vi "rmad skredstorrelse.vi"(0 "Is Logging":T5(array[cluster]), 1 "State":u16(ring) items=["Init", "Write"], 2 "Rød signal kriterie":bool[](array[boolean]), 5 "Avalanch Packets":T4(array[cluster]) {"A1 std" format="%.1f"; "A2 std" format="%.1f"; "A3 std" format="%.1g"; "A4 std" format="%.1g"}, 7 "Recent events":T1(array[cluster]) {"SPS" format="%.1f"}, 12 "Stredstørrelser terskelverdier":T2(array[cluster])) -> (4 "Skredhendelser":T3(array[cluster]) {"Intensitet terskel 1" format="%.1f"; "Intensitet terskel 2" format="%.1f"; "Intensitet terskel 3" format="%.1f"; "Intensitet terskel 4" format="%.1f"; "Intensitet terskel 5" format="%.1f"}, 6 "event to regobs":bool[](array[boolean]), 8 "event to file?":bool[](array[boolean]), 10 "is logging":bool[](array[boolean]), 14 "num pack pr size":u16[][](array[numeric]))   [LabVIEW 2017]
panel:
  out "har aktivert rødt lys":bool[](array[boolean])
  out "løpende gjennomsnitt":dbl[][](array[numeric])
  out "sum intensiteter":dbl[][](array[numeric])
  out "har trigget på denne event":bool[](array[boolean])
  out "skredstorelse index":i32[](array[numeric])
  out "packet number index":u16[](array[numeric])
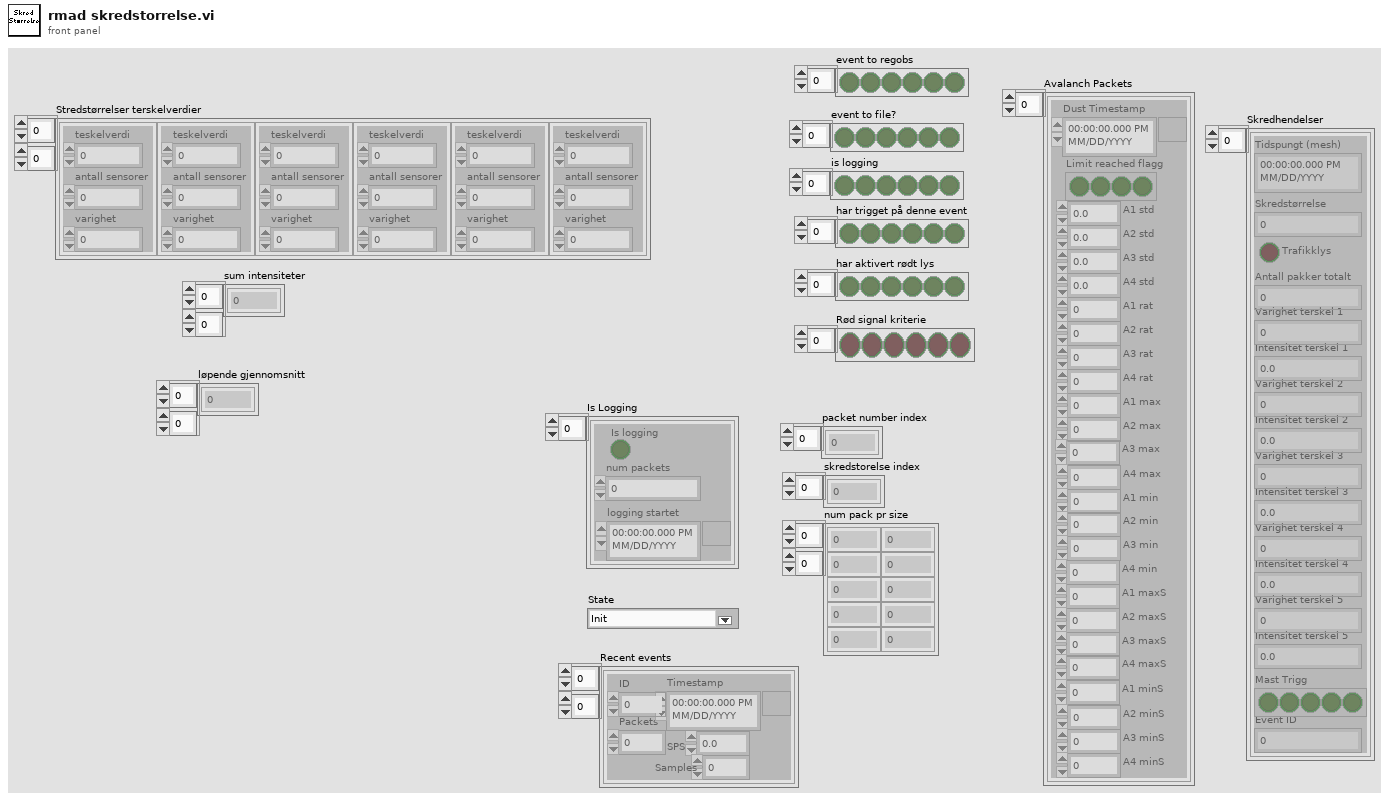
[diagram p1: front panel]
types:
  T1 = cluster{"ID":u16, "Timestamp":timestamp, "Packets":u16, "SPS":dbl, "Samples":u16}[][]
  T2 = cluster{"teskelverdi":u32, "antall sensorer":u32, "varighet":u32}[][]
  T3 = cluster{"Tidspungt (mesh)":timestamp, "Skredstørrelse":u16, "Trafikklys":bool, "Antall pakker totalt":u16, "Varighet terskel 1":u16, "Intensitet terskel 1":dbl, "Varighet terskel 2":u16, "Intensitet terskel 2":dbl, "Varighet terskel 3":u16, "Intensitet terskel 3":dbl, "Varighet terskel 4":u16, "Intensitet terskel 4":dbl, "Varighet terskel 5":u16, "Intensitet terskel 5":dbl, "Mast Trigg":bool[], "Event ID":i32}[]
  T4 = cluster{"Dust Timestamp":timestamp, "Limit reached flagg":bool[], "A1 std":sgl, "A2 std":sgl, "A3 std":sgl, "A4 std":sgl, "A1 rat":sgl, "A2 rat":sgl, "A3 rat":sgl, "A4 rat":sgl, "A1 max":u16, "A2 max":u16, "A3 max":u16, "A4 max":u16, "A1 min":u16, "A2 min":u16, "A3 min":u16, "A4 min":u16, "A1 maxS":u16, "A2 maxS":u16, "A3 maxS":u16, "A4 maxS":u16, "A1 minS":u16, "A2 minS":u16, "A3 minS":u16, "A4 minS":u16}[]
  T5 = cluster{"Is logging":bool, "num packets":u16, "logging startet":timestamp}[]
  T6 = cluster{"logging startet":timestamp, i32, bool, "num packets":u16, u16, dbl, u16, dbl, u16, dbl, u16, dbl, u16, dbl, bool[], "index":i32}
  T7 = cluster{"ID":u16, "Timestamp":timestamp, "Packets":u16, "SPS":dbl, "Samples":u16}
  T8 = cluster{"logging startet":timestamp, i32, bool, "num packets":u16, u16, dbl, u16, dbl, "index":i32, "index":i32, "index":i32, "index":i32, "index":i32, "index":i32, bool[], "ID":u16}
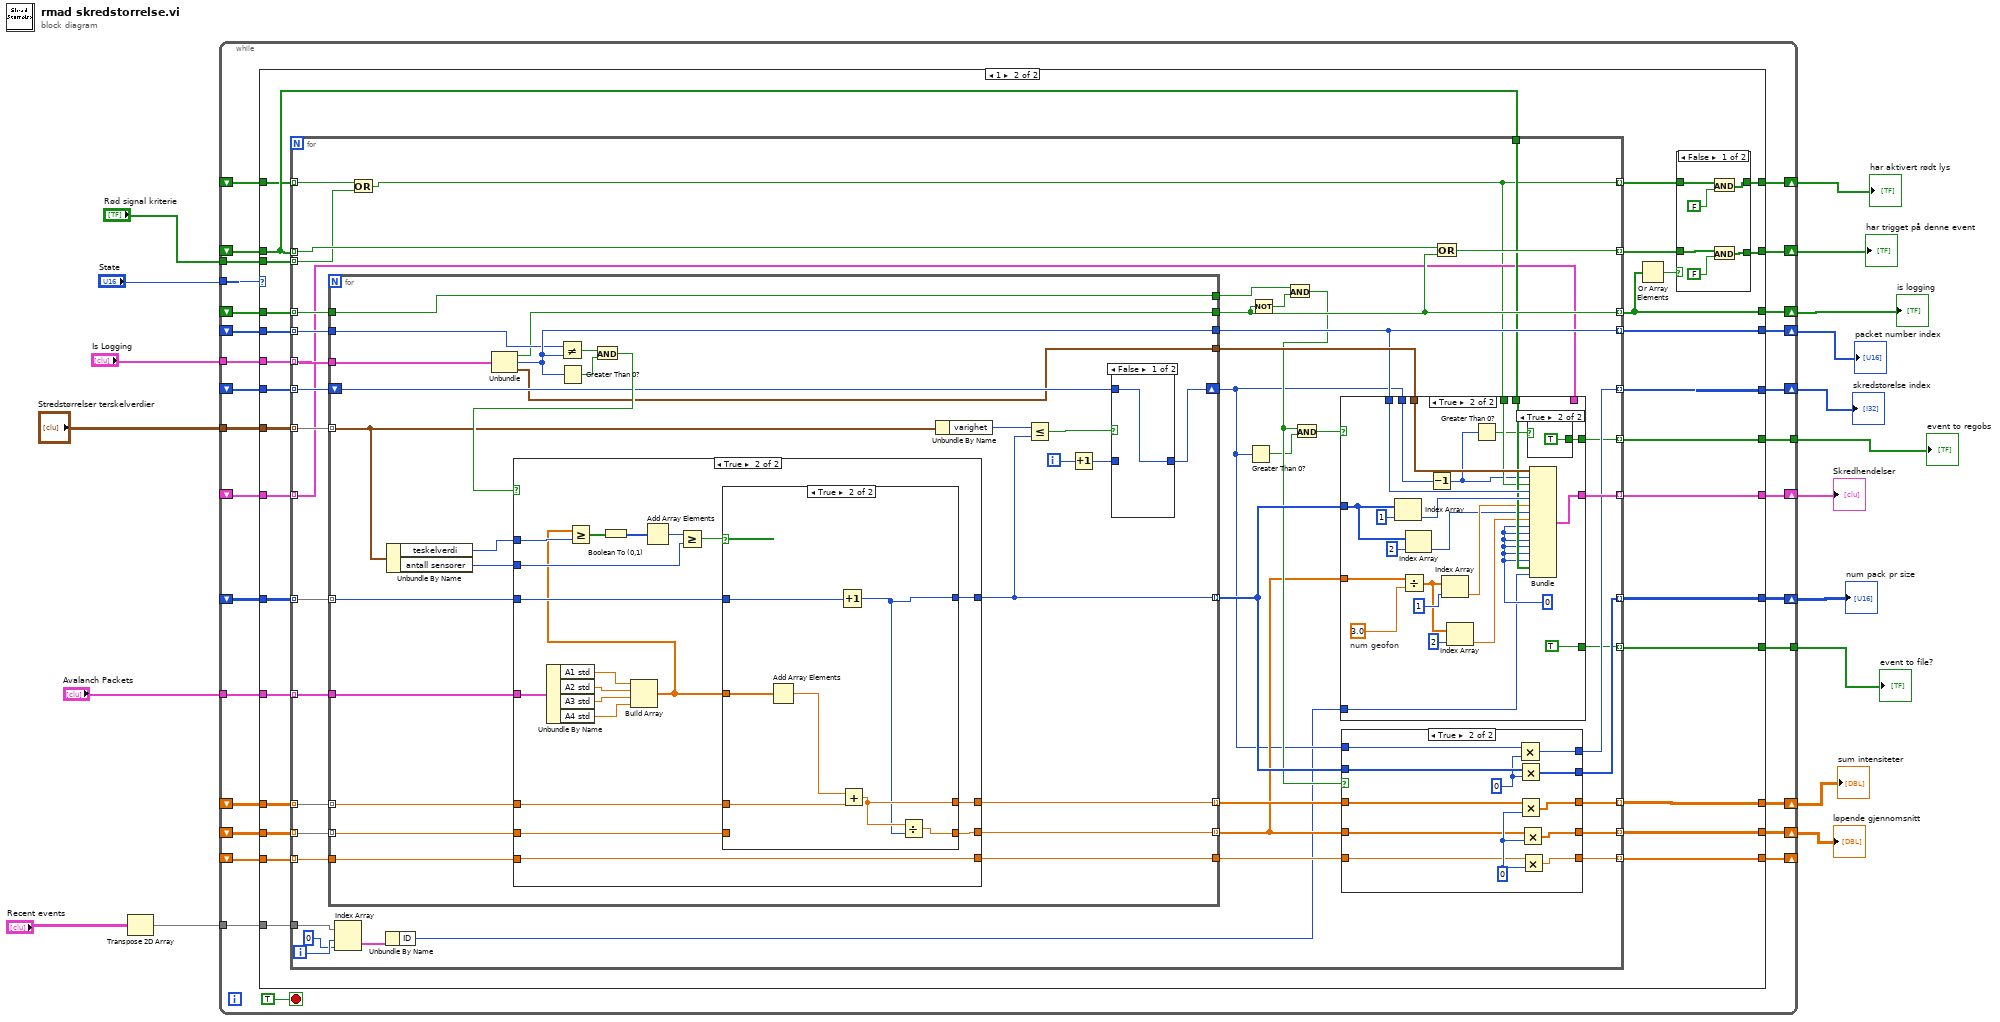
[diagram p0: block diagram]
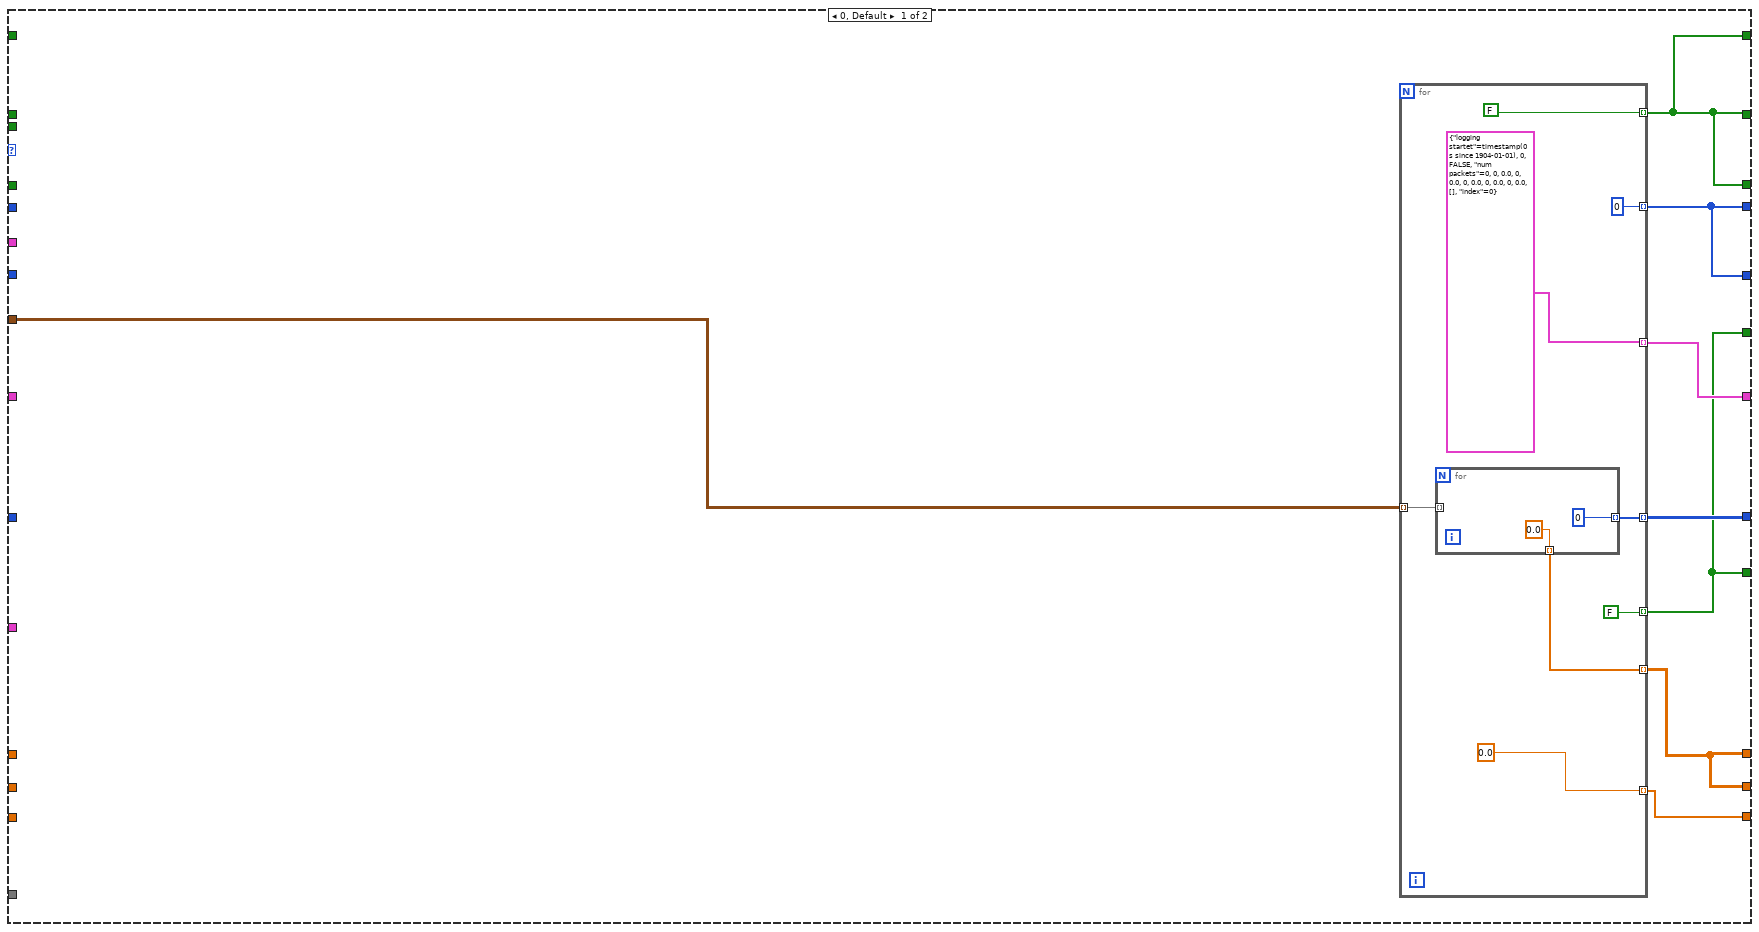
[diagram p2: hidden frame]
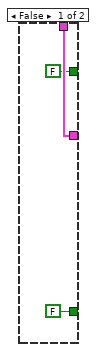
[diagram p5: hidden frame]
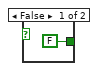
[diagram p6: hidden frame]
diagram:
  n1 = Transpose 2D Array(2D array="Recent events") -> (transposed array=w4:T1)
  n2 = while {
    tunnel: "Is Logging" -> [w47]
    tunnel: "Avalanch Packets" -> [w45]
    tunnel: "State" -> [w44]
    tunnel: "Stredstørrelser terskelverdier" -> [w43]
    shift-right: [w42] -> w11
    shift-left: _ -> [w41]
    shift-right: [w40] -> w15
    shift-left: _ -> [w39]
    shift-right: [w38] -> w14
    shift-left: _ -> [w37]
    shift-right: [w36] -> _
    shift-left: _ -> [w33]
    shift-right: [w35] -> w8
    shift-left: _ -> [w32]
    shift-right: [w34] -> w10
    shift-left: _ -> [w31]
    shift-right: [w30] -> w13
    shift-left: _ -> [w29]
    shift-right: [w28] -> w12
    shift-left: _ -> [w27]
    shift-right: [w26] -> w9
    shift-left: _ -> [w25]
    tunnel: [w24] -> w6
    tunnel: "Rød signal kriterie" -> [w23]
    tunnel: w4 -> [w22]
    tunnel: [w21] -> w2
    shift-right: [w20] -> w1
    shift-left: _ -> [w19]
    stop <- TRUE stop-if-true
    n3 = case shown="1" w44 {
      tunnel: w47 -> [_ w95]
      tunnel: w45 -> [_ w94]
      tunnel: w43 -> [w54 w93]
      tunnel: [w53 w92] -> w42
      tunnel: w41 -> [_ w91]
      tunnel: [w55 w90] -> w40
      tunnel: w39 -> [_ w89]
      tunnel: [w55 w88] -> w38
      tunnel: w37 -> [_ w87]
      tunnel: [w51 w86] -> w36
      tunnel: [w50 w85] -> w35
      tunnel: [w50 w84] -> w34
      tunnel: w33 -> [_ w83]
      tunnel: w32 -> [_ w82]
      tunnel: w31 -> [_ w81]
      tunnel: [w48 w79] -> w30
      tunnel: w29 -> [_ w80]
      tunnel: [w48 w77] -> w28
      tunnel: w27 -> [_ w75]
      tunnel: [w52 w74] -> w26
      tunnel: w25 -> [_ w73]
      tunnel: [w49 w72] -> w24
      tunnel: w23 -> [_ w71]
      tunnel: w22 -> [_ w70]
      tunnel: [w49 w69] -> w21
      tunnel: [w48 w66] -> w20
      tunnel: w19 -> [_ w68]
      frame 0, Default {
        n4 = for {
          tunnel: [u16 0] -> w55 mode=indexing
          tunnel: [FALSE] -> w48 mode=indexing
          tunnel: [0.0 ("number")] -> w51 mode=indexing
          tunnel: w54 -> [w60] mode=indexing
          tunnel: [w59] -> w53 mode=indexing
          tunnel: [T6 {"logging startet"=timestamp(0 s since 1904-01-01), 0, FALSE, "num packets"=0, 0, 0.0, 0, 0.0, 0, 0.0, 0, 0.0, 0, 0.0, [], "index"=0}] -> w52 mode=indexing
          tunnel: [w58] -> w50 mode=indexing
          tunnel: [FALSE] -> w49 mode=indexing
          n5 = for {
            tunnel: w60 -> [_] mode=indexing
            tunnel: [u16 0] -> w59 mode=indexing
            tunnel: [0.0 ("number")] -> w58 mode=indexing
          }
        }
      }
      frame 1 {
        n6 = for {
          tunnel: w95 -> [w145] mode=indexing
          tunnel: w94 -> [w146] mode=indexing
          tunnel: w93 -> [w144] mode=indexing
          tunnel: [w122] -> w92 mode=indexing
          tunnel: w91 -> [w143] mode=indexing
          tunnel: [w133] -> w90 mode=indexing
          tunnel: w89 -> [w142] mode=indexing
          tunnel: [w116] -> w88 mode=indexing
          tunnel: w87 -> [w141] mode=indexing
          tunnel: [w125] -> w86 mode=indexing
          tunnel: [w124] -> w85 mode=indexing
          tunnel: [w123] -> w84 mode=indexing
          tunnel: w83 -> [w140] mode=indexing
          tunnel: w82 -> [w139] mode=indexing
          tunnel: w81 -> [w138] mode=indexing
          tunnel: [w132] -> w79 mode=indexing
          tunnel: w80 -> [w137] mode=indexing
          tunnel: [w131] -> w78 mode=indexing
          tunnel: w75 -> [w130] mode=indexing
          tunnel: w75 -> [w129]
          tunnel: [w128] -> w74 mode=indexing
          tunnel: w73 -> [w127] mode=indexing
          tunnel: [w114] -> w72 mode=indexing
          tunnel: w71 -> [w105] mode=indexing
          tunnel: w70 -> [w113]
          tunnel: [w107] -> w69 mode=indexing
          tunnel: w68 -> [w106] mode=indexing
          tunnel: [w104] -> w67 mode=indexing
          i -> [w110]
          n7 = for {
            tunnel: w146 -> [w218]
            tunnel: w145 -> [w215]
            tunnel: w144 -> [w209] mode=indexing
            tunnel: [w195] -> w126 mode=indexing
            tunnel: w143 -> [w214] mode=indexing
            tunnel: [w211] -> w133
            tunnel: w142 -> [w210]
            shift-right: [w204] -> w117
            shift-left: w141 -> [w203]
            tunnel: [w202] -> w121
            tunnel: [w201] -> w118 mode=indexing
            tunnel: [w200] -> w119 mode=indexing
            tunnel: w140 -> [w199]
            tunnel: w139 -> [w198] mode=indexing
            tunnel: w138 -> [w197] mode=indexing
            tunnel: [w196] -> w132
            tunnel: w137 -> [w194]
            tunnel: [w194] -> w135
            tunnel: [w193] -> w134
            i -> [w206]
            n8 = Unbundle By Name(w209) -> ("teskelverdi"=w216:u32, "antall sensorer"=w217:u32)
            n9 = Unbundle(w215) -> ("Is logging"=w196:bool, "num packets"=w211:u16, "logging startet"=w193:timestamp)
            n10 = Not Equal?(x=w210, y=w211) -> (x != y?=w219:bool)
            n11 = Greater Than 0?(x=w211) -> (x > 0?=w213:bool)
            n12 = And(x=w219, y=w213) -> (x .and. y?=w212:bool)
            n13 = case shown="True" w212 {
              tunnel: w218 -> [_ w244]
              tunnel: w217 -> [_ w234]
              tunnel: w216 -> [_ w235]
              tunnel: [w225 w233] -> w195
              tunnel: w214 -> [w225 w232]
              tunnel: [w222 w230] -> w202
              tunnel: [w223 w227] -> w201
              tunnel: [w224 w228] -> w200
              tunnel: w199 -> [w222 w230]
              tunnel: w198 -> [w223 w226]
              tunnel: w197 -> [w224 w229]
              frame False {
              }
              frame True {
                n14 = Unbundle By Name(w244) -> ("A1 std"=w242:sgl, "A2 std"=w243:sgl, "A3 std"=w241:sgl, "A4 std"=w240:sgl)
                n15 = Build Array(w242, w243, w241, w240) -> (w231:sgl[])
                n16 = Greater Or Equal?(x=w231, y=w235) -> (x >= y?=w239:bool[])
                n17 = Boolean To (0,1)(Boolean=w239) -> (0, 1=w238:i16[])
                n18 = Add Array Elements(numeric array=w238) -> (sum=w237:i16)
                n19 = Greater Or Equal?(x=w237, y=w234) -> (x >= y?=w236:bool)
                n20 = case shown="True" w236 {
                  tunnel: [w247 w249] -> w233
                  tunnel: w232 -> [w247 w254]
                  tunnel: w231 -> [_ w253]
                  tunnel: w229 -> [w246 w252]
                  tunnel: [w246 w250] -> w228
                  tunnel: [w245 w248] -> w227
                  tunnel: w226 -> [w245 _]
                  frame False {
                  }
                  frame True {
                    n21 = Add Array Elements(numeric array=w253) -> (sum=w251:sgl)
                    n22 = Increment(x=w254) -> (x+1=w249:u16)
                    n23 = Add(x=w251, y=w252) -> (x+y=w250:dbl)
                    n24 = Divide(x=w250, y=w249) -> (x/y=w248:dbl)
                  }
                }
              }
            }
            n25 = Unbundle By Name(w209) -> ("varighet"=w208:u32)
            n26 = Less Or Equal?(x=w208, y=w195) -> (x <= y?=w207:bool)
            n27 = Increment(x=w206) -> (x+1=w205:i32)
            n28 = case shown="False" w207 {
              tunnel: w205 -> [_ w221]
              tunnel: [w220 w221] -> w204
              tunnel: w203 -> [w220 _]
              frame False {
              }
              frame True {
              }
            }
          }
          n29 = Index Array(array=w113, index (row)=w110, index (col)=0 ("index")) -> (element=w112:T7)
          n30 = Or(x=w106, y=w105) -> (x .or. y?=w104:bool)
          n31 = Unbundle By Name(w112) -> ("ID"=w111:u16)
          n32 = Greater Than 0?(x=w117) -> (x > 0?=w108:bool)
          n33 = Not(x=w132) -> (.not. x?=w136:bool)
          n34 = And(x=w135, y=w136) -> (x .and. y?=w120:bool)
          n35 = And(x=w120, y=w108) -> (x .and. y?=w115:bool)
          n36 = case shown="True" w115 {
            tunnel: w134 -> [_ w190]
            tunnel: w133 -> [_ w189]
            tunnel: w117 -> [_ w170]
            tunnel: w129 -> [_ w181]
            tunnel: [w166 w185] -> w128
            tunnel: w127 -> [w166 _]
            tunnel: w126 -> [_ w183]
            tunnel: w118 -> [_ w174]
            tunnel: [FALSE TRUE] -> w114
            tunnel: w104 -> [_ w172]
            tunnel: w111 -> [_ w171]
            tunnel: [FALSE w167] -> w107
            frame False {
            }
            frame True {
              w175 = 0 ("index")
              w184 = 3.0  # num geofon
              n37 = Index Array(array=w183, index=1) -> (element=w186:u16)
              n38 = Divide(x=w174, y=w184) -> (x/y=w177:dbl[])
              n39 = Index Array(array=w183, index=2) -> (element=w179:u16)
              n40 = Decrement(x=w170) -> (x-1=w169:i32)
              n41 = Index Array(array=w177, index=1) -> (element=w180:dbl)
              n42 = Index Array(array=w177, index=2) -> (element=w176:dbl)
              n43 = Greater Than 0?(x=w169) -> (x > 0?=w168:bool)
              n44 = case shown="True" w168 {
                tunnel: [FALSE TRUE] -> w167
                frame False {
                }
                frame True {
                }
              }
              n45 = Bundle("logging startet"=w190, w169, w172, "num packets"=w189, w186, w180, w179, w176, "index"=w175, "index"=w175, "index"=w175, "index"=w175, "index"=w175, "index"=w175, w181, "ID"=w171) -> (w185:T8)  [unwired: 1 in]
            }
          }
          n46 = case shown="True" w120 {
            tunnel: w126 -> [w151 w156]
            tunnel: w119 -> [w150 w162]
            tunnel: w118 -> [w149 w161]
            tunnel: w121 -> [w148 w160]
            tunnel: [w148 w159] -> w125
            tunnel: [w149 w158] -> w124
            tunnel: [w150 w157] -> w123
            tunnel: [w151 w155] -> w122
            tunnel: w117 -> [w147 w154]
            tunnel: [w147 w152] -> w116
            frame False {
            }
            frame True {
              w153 = u16 0
              w163 = u16 0
              n47 = Multiply(x=w154, y=w153) -> (x*y=w152:i32)
              n48 = Multiply(x=w156, y=w153) -> (x*y=w155:u16[])
              n49 = Multiply(x=w162, y=w163) -> (x*y=w157:dbl[])
              n50 = Multiply(x=w161, y=w163) -> (x*y=w158:dbl[])
              n51 = Multiply(x=w160, y=w163) -> (x*y=w159:dbl)
            }
          }
          n52 = Or(x=w130, y=w132) -> (x .or. y?=w131:bool)
        }
        n53 = Or Array Elements(Boolean array=w79) -> (logical OR=w76:bool)
        n54 = case shown="False" w76 {
          tunnel: w78 -> [w101 w103]
          tunnel: [w100 w103] -> w77
          tunnel: w67 -> [w97 w102]
          tunnel: [w96 w102] -> w66
          frame False {
            n55 = And(x=w97, y=FALSE) -> (x .and. y?=w96:bool[])
            n56 = And(x=w101, y=FALSE) -> (x .and. y?=w100:bool[])
          }
          frame True {
          }
        }
      }
    }
  }
  "packet number index" <- w15
  "skredstorelse index" <- w14
  "is logging" <- w13
  "har trigget på denne event" <- w12
  "num pack pr size" <- w11
  "sum intensiteter" <- w10
  "Skredhendelser" <- w9
  "løpende gjennomsnitt" <- w8
  "event to file?" <- w6
  "event to regobs" <- w2
  "har aktivert rødt lys" <- w1
